vi "Write position.vi"(8 "error in (no error)":errorcluster, 10 "position":cluster{"x":dbl, "y":dbl}[](array[cluster]), 11 "Snake in":refnum<class "Snake.lvclass">) -> (0 "error out":errorcluster, 3 "Snake out":refnum<class "Snake.lvclass">)   [LabVIEW 2021]
uses:
  Snake.lvclass
  C:/Users/poche/Programs/LabVIEW/imposible snake/GameEl_class/GameEl.lvclass
  GameEl_class/GameEl.lvclass/GameEl.ctl
  GameEl_class/GameEl.lvclass
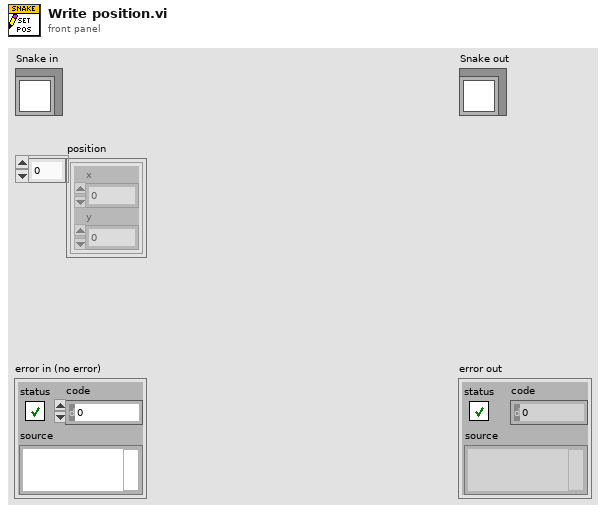
[diagram p1: front panel]
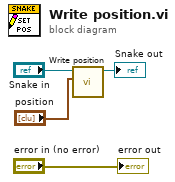
[diagram p0: block diagram]
diagram:
  n1 = call "Write position.vi"("position"="position", "GameEl in"="Snake in") -> ("GameEl out"=→"Snake out":refnum<class "Snake.lvclass">)  [unwired: 8 in, 1 out]
  "error out" <- "error in (no error)"
